vi "search_peak_xrf.vi"(9 "width":i32=20 min=3, 10 "threshold":dbl=20.0 format="%0.2f", 11 "data_test":T1={"Array"=array[8192 elements], "Spectrum - Background"=array[8192 elements]}) -> (1 "Best 8":i32[][](array[numeric])=[[9, 8, 47, 4, 36, 35, 48, 28], [4, 4, 14, 3, 12, 12, 12, 12]], 2 "peaks found":i32=60, 3 "set max":cluster{"Channels":dbl[], "Intensity":dbl[]}={"Channels"=[0.6846487923218129, 0.8031614293624534, 1.7242543828557408, 1.938747247460668, 2.306953300257028, 2.6210970168759666, 2.9711981229526625, 3.3277824164248653, 3.7170873790620336, 4.04405224728037, 6.436481431667202, 7.096967343713246, 7.460990586502177, 7.523333804369678, 7.617042760860395, 8.127017296174136, 8.194901838112248, 8.297705547082785, 8.30569855209705, 8.683571266368165, 9.291525652441827, 9.336316527839342, 9.702473642891427, 10.164949159251092, 10.940151266361038, 10.984300604976537, 11.073242471735028, 11.160271165263742, 11.268603021790387, 11.368683422279902, 11.476870860603926, 11.732338216351955, 11.74047488132859, 11.913527841198139, 12.313442472513525, 12.422414883693174, 12.679357859240612, 13.137181465596367, 13.560377222755834, 13.985871403462042, 14.181757913002619, 14.811990689785183, 15.123878999537014, 15.225144239474576, 15.847402751701654, 15.936506376474796, 15.997115442383588, 16.751668923733696, 17.456338945421972, 18.685517095107702, 19.565242039112338, 23.10994450808025, 23.25953036719509, 23.37377015691927, 23.439242722748002, 23.98629158276466, 24.428149293414577, 24.684829964850557, 24.772035910147434, 25.173301655535283], "Intensity"=[5749.475271060954, 5002.0142432044795, 4437.978004734703, 11660.526656612647, 65746.84001208292, 2894.387213953257, 9849.360532927198, 7160.035072829482, 645601.7858592308, 95492.33538323875, 14805.060779816191, 1620.7095092057602, 1146.3915335122922, 1168.4930336372568, 1322.5033864359928, 4245.563045439152, 4184.35157964611, 4422.765014063421, 4401.872906279167, 13740.871473164421, 12716.350040257696, 12964.336303896753, 16789.033949154484, 20702.823823277406, 27073.790223214626, 26827.13611017004, 26877.36292640188, 26681.744011808405, 26623.286988764616, 26394.35650952068, 26015.737537837078, 23980.0092551179, 23996.924012643343, 23101.773776484937, 20651.803398511016, 20229.386024779047, 41284.21044656313, 13637.881570622103, 8980.093476318705, 5646.466867551864, 7355.058688359613, 4885.822952660352, 292.0377308174795, 694.6108290767994, 6797.9436035222725, 6852.18604910736, 6738.9197496309225, 156943.61193784876, 77075.8593535495, 10701.96206664513, 3415.986171238152, 30.039025289396076, 37.780232933378514, 78.71549190995782, 52.215114100379424, 895.4437472888932, 1309.544166875224, 1288.517058471017, 1383.105839373177, 18123.868845544213]})   [LabVIEW 2023]
uses:
  <vilib>/Analysis/1siggen.llb/Ramp Pattern by Samples.vi
  <vilib>/Analysis/NI_AAL_SigProc.lvlib
  <vilib>/Analysis/NI_AALBase.lvlib
  <vilib>/Analysis/NI_AALPro.lvlib
panel:
  out "transposed array":i32[][](array[numeric])=[[9, 8, 47, 4, 36, 35, 48, 28, 27, 29, 26, 30, 25, 34, 24, 31, 32, 33, 46, 43, 18, 17, 39, 16, 15, 40, 11, 14, 13, 41, 12, 2, 10, 44, 23, 5, 22, 20, 1, 37, 0, 45, 6, 7, 19, 21, 38, 42, 49, 50, 51, 54, 52, 55, 57, 56, 53, 59, 58, 3], [4, 4, 14, 3, 12, 12, 12, 12, 12, 12, 12, 12, 12, 12, 12, 12, 12, 12, 11, 10, 8, 8, -224, 8, 7, -201, 7, 6, 6, -290, 6, -5, 6, -79, 10, -21794, 10, 4, -11, -1347, -11, -36, -5, 4, 9, 6, -3529, -1759, 19, 28, 508, 161, 291, 28, 29, 28, 86, 28, 28, -251]]
  out "subarray":i64[][](array[numeric])=[[4, 4, 14, 3, 12, 12, 12, 12], [23806, 23804, 21678, 14099, 13708, 13175, 12150, 11314]]
  out "Array":i64[][](array[numeric])=[[4, 4, 14, 3, 12, 12, 12, 12, 12, 12, 12, 12, 12, 12, 12, 12, 12, 12, 11, 10, 8, 8, -224, 8, 7, -201, 7, 6, 6, -290, 6, -5, 6, -79, 10, -21794, 10, 4, -11, -1347, -11, -36, -5, 4, 9, 6, -3529, -1759, 19, 28, 508, 161, 291, 28, 29, 28, 86, 28, 28, -251], [23806, 23804, 21678, 14099, 13708, 13175, 12150, 11314, 11285, 11272, 11179, 11175, 10971, 10919, 10858, 10782, 10769, 10562, 10084, 9637, 6818, 6803, 6726, 6683, 6672, 6543, 6422, 5659, 5465, 5316, 4608, 4505, 4501, 4372, 3809, 3002, 2629, 2349, 2042, 1833, 1608, 1559, 1558, 1130, 405, 286, 128, -1552, -2924, -5645, -7513, -9547, -10272, -17068, -17114, -17398, -17912, -18782, -18837, -43148]]
  out "XY Graph":cluster{"Locations":dbl[], "Amplitudes":dbl[]}[](graph)=[{"Locations"=array[8192 elements], "Amplitudes"=array[8192 elements]}, {"Locations"=[0.6846487923218129, 0.8031614293624534, 1.7242543828557408, 1.938747247460668, 2.306953300257028, 2.6210970168759666, 2.9711981229526625, 3.3277824164248653, 3.7170873790620336, 4.04405224728037, 6.436481431667202, 7.096967343713246, 7.460990586502177, 7.523333804369678, 7.617042760860395, 8.127017296174136, 8.194901838112248, 8.297705547082785, 8.30569855209705, 8.683571266368165, 9.291525652441827, 9.336316527839342, 9.702473642891427, 10.164949159251092, 10.940151266361038, 10.984300604976537, 11.073242471735028, 11.160271165263742, 11.268603021790387, 11.368683422279902, 11.476870860603926, 11.732338216351955, 11.74047488132859, 11.913527841198139, 12.313442472513525, 12.422414883693174, 12.679357859240612, 13.137181465596367, 13.560377222755834, 13.985871403462042, 14.181757913002619, 14.811990689785183, 15.123878999537014, 15.225144239474576, 15.847402751701654, 15.936506376474796, 15.997115442383588, 16.751668923733696, 17.456338945421972, 18.685517095107702, 19.565242039112338, 23.10994450808025, 23.25953036719509, 23.37377015691927, 23.439242722748002, 23.98629158276466, 24.428149293414577, 24.684829964850557, 24.772035910147434, 25.173301655535283], "Amplitudes"=[5749.475271060954, 5002.0142432044795, 4437.978004734703, 11660.526656612647, 65746.84001208292, 2894.387213953257, 9849.360532927198, 7160.035072829482, 645601.7858592308, 95492.33538323875, 14805.060779816191, 1620.7095092057602, 1146.3915335122922, 1168.4930336372568, 1322.5033864359928, 4245.563045439152, 4184.35157964611, 4422.765014063421, 4401.872906279167, 13740.871473164421, 12716.350040257696, 12964.336303896753, 16789.033949154484, 20702.823823277406, 27073.790223214626, 26827.13611017004, 26877.36292640188, 26681.744011808405, 26623.286988764616, 26394.35650952068, 26015.737537837078, 23980.0092551179, 23996.924012643343, 23101.773776484937, 20651.803398511016, 20229.386024779047, 41284.21044656313, 13637.881570622103, 8980.093476318705, 5646.466867551864, 7355.058688359613, 4885.822952660352, 292.0377308174795, 694.6108290767994, 6797.9436035222725, 6852.18604910736, 6738.9197496309225, 156943.61193784876, 77075.8593535495, 10701.96206664513, 3415.986171238152, 30.039025289396076, 37.780232933378514, 78.71549190995782, 52.215114100379424, 895.4437472888932, 1309.544166875224, 1288.517058471017, 1383.105839373177, 18123.868845544213]}]
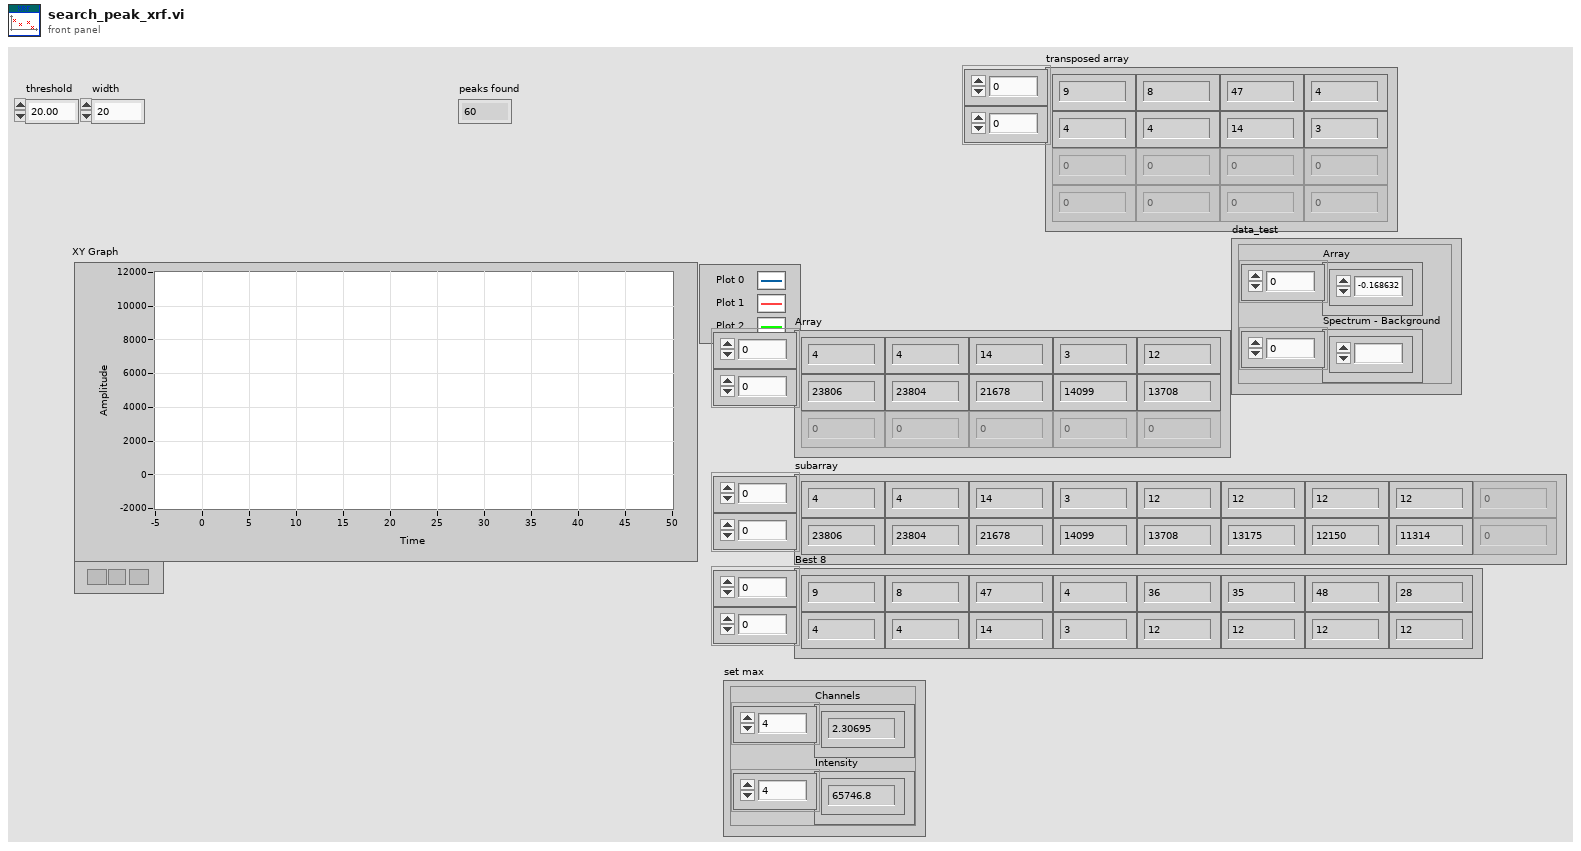
[diagram p1: front panel]
types:
  T1 = cluster{"Array":dbl[], "Spectrum - Background":dbl[]}
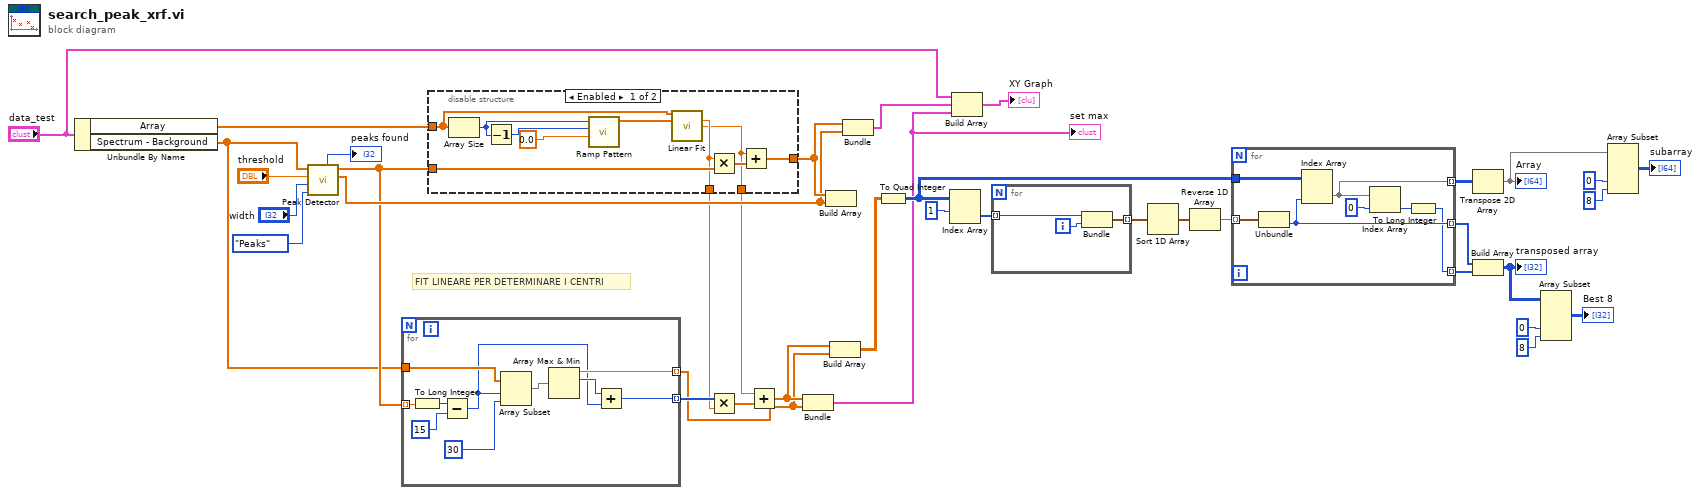
[diagram p0: block diagram]
diagram:
  # "FIT LINEARE PER DETERMINARE I CENTRI"
  n1 = Unbundle By Name("data_test") -> ("Array"=w10:dbl[], "Spectrum - Background"=w9:dbl[])
  n2 = call <vilib>:"Peak Detector.vi"("peaks/valleys"=enum32{"Peaks", "Valleys"}."Peaks", "width"="width", "threshold"="threshold", "X"=w9) -> ("Amplitudes"=w12:dbl[], "Locations"=w11:dbl[], "# found"=→"peaks found":i32)  [unwired: 3 in, 2 out]
  n3 = for {
    tunnel: w9 -> [w44]
    tunnel: w11 -> [w39] mode=indexing
    tunnel: [w42] -> w3 mode=indexing
    tunnel: [w40] -> w8 mode=indexing
    n4 = To Long Integer(number=w39) -> (32bit integer=w46:i32)
    n5 = Subtract(x=w46, y=15) -> (x-y=w38:i32)
    n6 = Array Subset(array=w44, index=w38, length=30) -> (w43:dbl[])
    n7 = Array Max & Min(array=w43) -> (max value=w42:dbl, max index (indices)=w41:i32)  [unwired: 2 out]
    n8 = Add(x=w41, y=w38) -> (x+y=w40:i32)
  }
  n9 = disable-structure shown="Enabled" {
    disable-tunnel: w10 -> [w54 _]
    disable-tunnel: w11 -> [w52 w58]
    disable-tunnel: [w50 w58] -> w13
    disable-tunnel: [w49 _] -> w7
    disable-tunnel: [w48 _] -> w5
    frame Enabled {
      n10 = Array Size(array=w54) -> (size(s)=w55:i32)
      n11 = Decrement(x=w55) -> (x-1=w56:i32)
      n12 = call-poly <vilib>:"Ramp Pattern.vi"("start"=0.0, "end"=w56, "samples"=w55) -> ("Ramp Pattern"=w53:dbl[])  [unwired: 7 in, 1 out]
      n13 = call <vilib>:"Linear Fit.vi"("Y"=w54, "X"=w53) -> ("slope"=w49:dbl, "intercept"=w48:dbl)  [unwired: 9 in, 3 out]
      n14 = Multiply(x=w49, y=w52) -> (x*y=w51:dbl[])
      n15 = Add(x=w48, y=w51) -> (x+y=w50:dbl[])
    }
    frame Disabled {
    }
  }
  n16 = Multiply(x=w8, y=w7) -> (x*y=w6:dbl[])
  n17 = Add(x=w5, y=w6) -> (x+y=w4:dbl[])
  n18 = Bundle(w4, w3) -> (w1:cluster{dbl[], dbl[]})  [unwired: 1 in]
  "set max" <- w1
  n19 = Build Array(w13, w12) -> ()  [unwired: 1 out]
  n20 = Build Array(w4, w3) -> (w2:dbl[][])
  n21 = Bundle(w13, "Amplitudes"=w12) -> (w14:cluster{dbl[], "Amplitudes":dbl[]})  [unwired: 1 in]
  n22 = To Quad Integer(1:w2) -> (0:w22:i64[][])
  n23 = Index Array(array=w22, index (row)=1 ("index")) -> (element=w29:i64[])  [unwired: 1 in]
  n24 = Build Array("data_test", w14, w1) -> (→"XY Graph":cluster{"Array":dbl[], "Amplitudes":dbl[]}[])
  n25 = for {
    tunnel: [w60] -> w32 mode=indexing
    tunnel: w29 -> [w59] mode=indexing
    i -> [w61]
    n26 = Bundle(w59, w61) -> (w60:cluster{i64, i32})  [unwired: 1 in]
  }
  n27 = Sort 1D Array(array=w32) -> (sorted array=w31:cluster{i64, i32}[])
  n28 = Reverse 1D Array(array=w31) -> (reversed array=w30:cluster{i64, i32}[])
  n29 = for {
    tunnel: w30 -> [w68] mode=indexing
    tunnel: w22 -> [w67]
    tunnel: [w65] -> w27 mode=indexing
    tunnel: [w66] -> w21 mode=indexing
    tunnel: [w62] -> w20 mode=indexing
    n30 = Unbundle(w68) -> (w66:i32)  [unwired: 1 out]
    n31 = Index Array(array=w67, index (col)=w66) -> (element=w65:i64[])  [unwired: 1 in]
    n32 = Index Array(array=w65, index=0) -> (element=w63:i64)
    n33 = To Long Integer(number=w63) -> (32bit integer=w62:i32)
  }
  n34 = Transpose 2D Array(2D array=w27) -> (transposed array=w26:i64[][])
  "Array" <- w26
  n35 = Build Array(w21, w20) -> (w17:i32[][])
  "transposed array" <- w17
  n36 = Array Subset(array=w17, index (col)=0 ("index"), length (col)=8 ("length")) -> (→"Best 8":i32[][])  [unwired: 2 in]
  n37 = Array Subset(array=w26, index (col)=0 ("index"), length (col)=8 ("length")) -> (→"subarray":i64[][])  [unwired: 2 in]
